vi "Multi-User Login.vi"() -> ()   [LabVIEW 2020]
uses:
  <vilib>/regexp/Match Regular Expression.xnode
panel:
  out "Error":string
  in  "AddButton":bool
  in  "New pass":string
  in  "New user":string
  out "Login status:":string
  out "Logged in":bool
  in  "LoginButton":bool
  in  "Password":string
  in  "Username":string
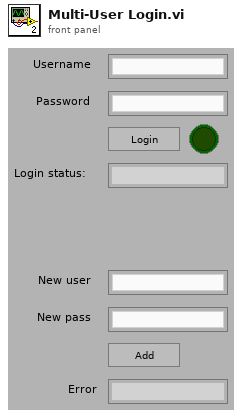
[diagram p1: front panel]
types:
  T1 = enum16{"open", "replace", "create", "open or create", "replace or create", "replace or create with confirmation"}
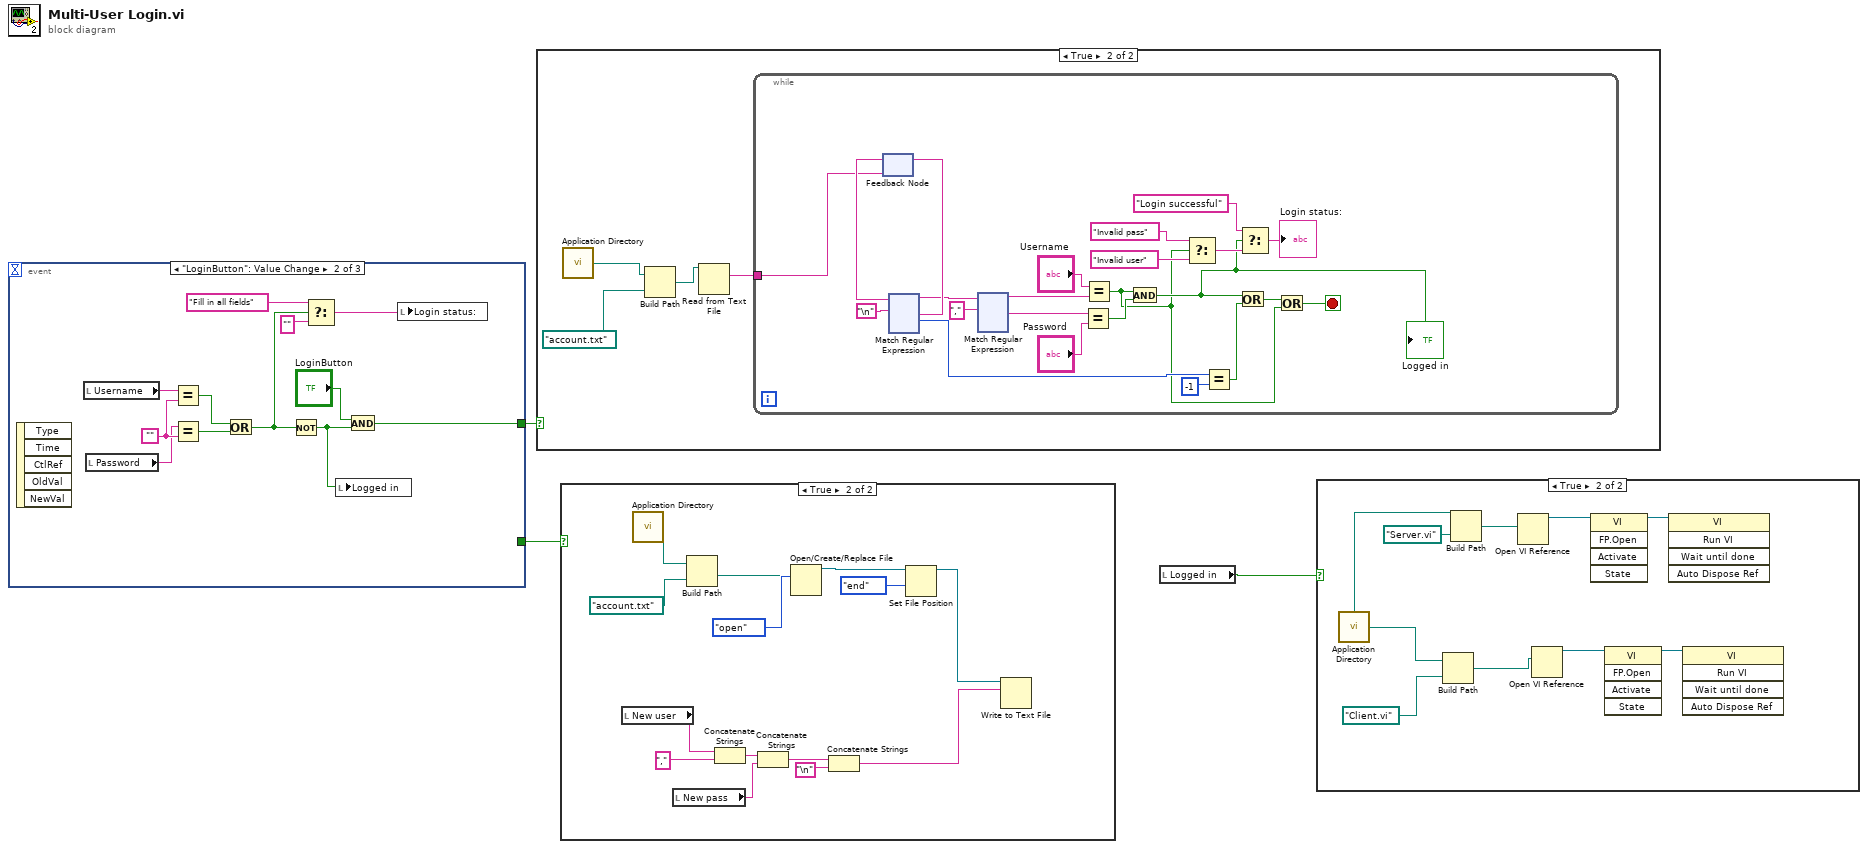
[diagram p0: block diagram]
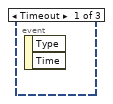
[diagram p5: hidden frame]
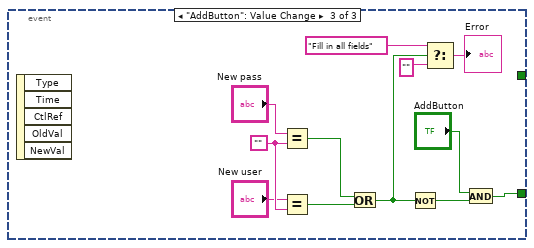
[diagram p6: hidden frame]
diagram:
  n1 = event shown="[1] \"LoginButton\": Value Change" {
    selector: _ -> [_ _ _]
    dyn-events: _ -> [_ _ _]
    timeout: _ -> [_ _ _]
    tunnel: [_ w14 _] -> w3
    tunnel: [_ _ w22] -> w2
    event Timeout {
      n2 = event-data() -> ()  [unwired: 1 in, 2 out]
    }
    event "LoginButton": Value Change {
      w9 = ""
      n3 = event-data() -> ()  [unwired: 1 in, 5 out]
      n4 = local read "Username"() -> (w10:string)
      n5 = local read "Password"() -> (w8:string)
      n6 = Equal?(x=w10, y=w9) -> (x = y?=w6:bool)
      n7 = Equal?(x=w8, y=w9) -> (x = y?=w7:bool)
      n8 = Or(x=w6, y=w7) -> (x .or. y?=w5:bool)
      n9 = Not(x=w5) -> (.not. x?=w4:bool)
      n10 = Select(t="Fill in all fields" ("regular expression"), s=w5, f="" ("regular expression")) -> (s? t:f=w13:string)
      n11 = local write "Logged in"(w4) -> ()
      n12 = And(x="LoginButton", y=w4) -> (x .and. y?=w14:bool)
      n13 = local write "Login status:"(w13) -> ()
    }
    event "AddButton": Value Change {
      w27 = ""
      n14 = event-data() -> ()  [unwired: 1 in, 5 out]
      n15 = Equal?(x="New pass", y=w27) -> (x = y?=w25:bool)
      n16 = Equal?(x="New user", y=w27) -> (x = y?=w26:bool)
      n17 = Or(x=w25, y=w26) -> (x .or. y?=w16:bool)
      n18 = Not(x=w16) -> (.not. x?=w17:bool)
      n19 = Select(t="Fill in all fields" ("regular expression"), s=w16, f="" ("regular expression")) -> (s? t:f=→"Error":string)
      n20 = And(x="AddButton", y=w17) -> (x .and. y?=w22:bool)
    }
  }
  n21 = case shown="True" w3 {
    frame False {
    }
    frame True {
      n22 = call <vilib>:"Application Directory.vi"() -> ("Application Directory"=w29:path)
      n23 = Build Path(base path=w29, name or relative path=path "account.txt") -> (appended path=w28:path)
      n24 = Read from Text File(file (use dialog)=w28) -> (text=w31:string)  [unwired: 3 in, 3 out]
      n25 = while {
        tunnel: w31 -> [w51]
        stop <- w32 stop-if-true
        n26 = feedback #1(w51) -> (w52:string)
        n27 = xnode "Match Regular Expression"("input string"=w52, "regular expression"="\n") -> ("before match"=w46:string, "after match"=w53:string, "offset past match"=w50:i32)  [unwired: 4 in, 2 out]
        n28 = feedback-in #1(w53) -> ()
        n29 = xnode "Match Regular Expression"("input string"=w46, "regular expression"=",") -> ("before match"=w44:string, "after match"=w43:string)  [unwired: 4 in, 3 out]
        n30 = Equal?(x=w43, y="Password") -> (x = y?=w40:bool)
        n31 = Equal?(x="Username", y=w44) -> (x = y?=w34:bool)
        n32 = And(x=w34, y=w40) -> (x .and. y?=w37:bool)
        "Logged in" <- w37
        n33 = Select(t="Invalid pass" ("regular expression"), s=w34, f="Invalid user" ("regular expression")) -> (s? t:f=w38:string)
        n34 = Equal?(x=w50, y=-1) -> (x = y?=w48:bool)
        n35 = Or(x=w37, y=w48) -> (x .or. y?=w33:bool)
        n36 = Select(t="Login successful" ("regular expression"), s=w37, f=w38) -> (s? t:f=→"Login status:":string)
        n37 = Or(x=w33, y=w34) -> (x .or. y?=w32:bool)
      }
    }
  }
  n38 = case shown="True" w2 {
    frame False {
    }
    frame True {
      n39 = local read "New user"() -> (w286:string)
      n40 = call <vilib>:"Application Directory.vi"() -> ("Application Directory"=w279:path)
      n41 = local read "New pass"() -> (w283:string)
      n42 = Build Path(base path=w279, name or relative path=path "account.txt") -> (appended path=w277:path)
      n43 = Concatenate Strings(w286, "," ("regular expression")) -> (w284:string)
      n44 = Concatenate Strings(w284, w283) -> (w282:string)
      n45 = Open/Create/Replace File(file path (use dialog)=w277, operation (0:open)=T1."open") -> (refnum out=w289:refnum<file>)  [unwired: 4 in, 2 out]
      n46 = Concatenate Strings(w282, "\n") -> (w280:string)
      n47 = Set File Position(refnum=w289, from (0:start)=enum16{"start", "end", "current"}."end") -> (refnum out=w287:refnum<file>)  [unwired: 2 in, 1 out]
      n48 = Write to Text File(file (use dialog)=w287, text=w280) -> ()  [unwired: 2 in, 3 out]
    }
  }
  n49 = local read "Logged in"() -> (w1:bool)
  n50 = case shown="True" w1 {
    frame False {
    }
    frame True {
      n51 = call <vilib>:"Application Directory.vi"() -> ("Application Directory"=w298:path)
      n52 = Build Path(base path=w298, name or relative path=path "Client.vi") -> (appended path=w291:path)
      n53 = Build Path(base path=w298, name or relative path=path "Server.vi") -> (appended path=w296:path)
      n54 = Open VI Reference(vi path=w296) -> (vi reference=w295:refnum<vi>)  [unwired: 5 in, 1 out]
      n55 = Open VI Reference(vi path=w291) -> (vi reference=w293:refnum<vi>)  [unwired: 5 in, 1 out]
      n56 = invoke class="VI" method="FP.Open"(reference=w295) -> (reference out=w294:refnum<vi>)  [unwired: 4 in, 4 out]
      n57 = invoke class="VI" method="FP.Open"(reference=w293) -> (reference out=w292:refnum<vi>)  [unwired: 4 in, 4 out]
      n58 = invoke class="VI" method="Run VI"(reference=w294) -> ()  [unwired: 4 in, 5 out]
      n59 = invoke class="VI" method="Run VI"(reference=w292) -> ()  [unwired: 4 in, 5 out]
    }
  }
